vi "Write Fire (%).vi"(8 "error in (no error)":errorcluster, 10 "Fire (%)":dbl format="%.2f", 11 "Oven Actor in":refnum<class "Oven Actor.lvclass">) -> (0 "error out":errorcluster, 3 "Oven Actor out":refnum<class "Oven Actor.lvclass">)   [LabVIEW 2024, in "Oven Actor.lvlib" / "Oven Actor.lvclass"]
uses:
  Oven Actor.lvclass
  Oven Actor.lvclass/Oven Actor.ctl
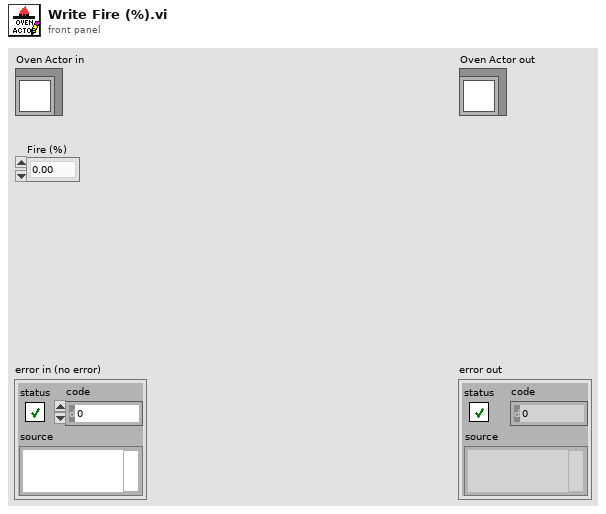
[diagram p1: front panel]
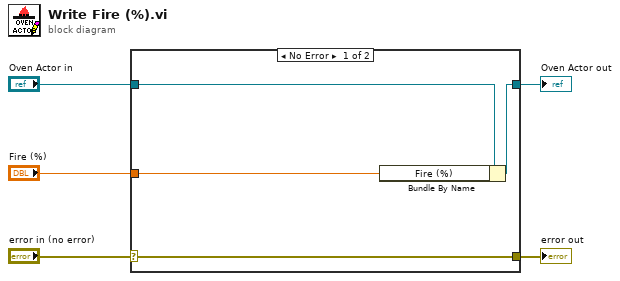
[diagram p0: block diagram]
diagram:
  n1 = case shown="No Error" "error in (no error)" {
    selector: "error in (no error)" -> [w9 w10]
    tunnel: [w9 w10] -> w4
    tunnel: [w7 w11] -> w2
    tunnel: "Oven Actor in" -> [w8 w11]
    tunnel: "Fire (%)" -> [w6 _]
    frame No Error {
      n2 = Bundle By Name(cluster=w8, "Fire (%)"=w6) -> (w7:refnum<class "Oven Actor.lvclass">)
    }
    frame Error {
    }
  }
  "error out" <- w4
  "Oven Actor out" <- w2
